vi "GetAllWatchdogs.vi"(8 "error in (no error)":errorcluster, 11 "Pound in":refnum<class "Pound.lvclass">) -> (0 "error out":errorcluster, 2 "All Watchdogs":refnum<data-value>[](array[refnum]), 3 "Pound out":refnum<class "Pound.lvclass">)   [LabVIEW 2017, in "Pound.lvclass"]
uses:
  <vilib>/NI/Software Watchdog/Pound/Pound.lvclass
  <vilib>/NI/Software Watchdog/Watchdog/Watchdog.lvclass
  <vilib>/NI/Software Watchdog/Pound/Pound.lvclass/Pound.ctl
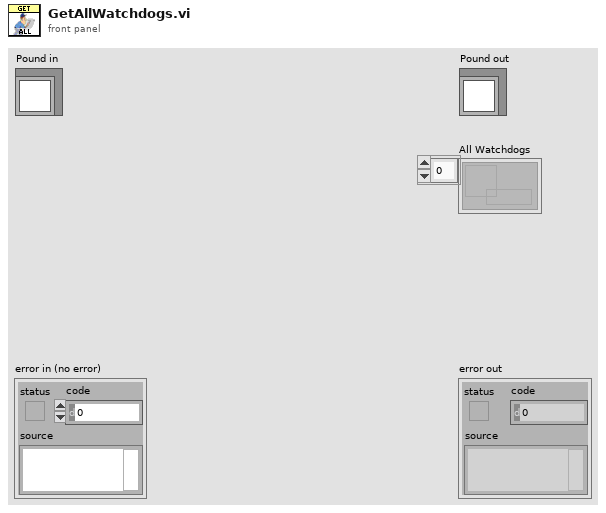
[diagram p1: front panel]
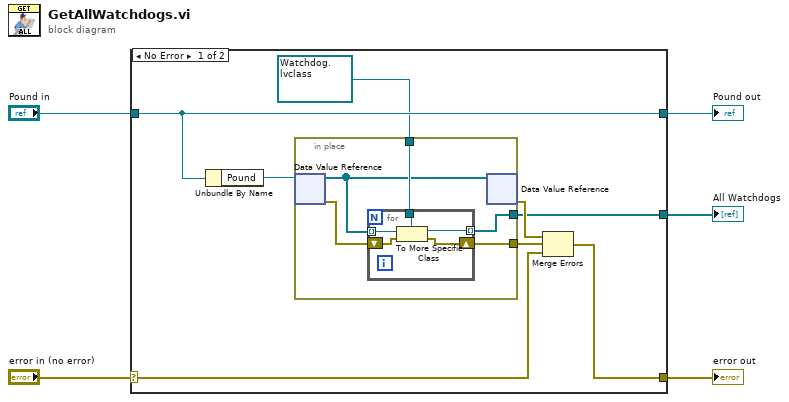
[diagram p0: block diagram]
diagram:
  n1 = case shown="No Error" "error in (no error)" {
    selector: "error in (no error)" -> [w6 w25]
    tunnel: [w8 w25] -> w4
    tunnel: [w12 w24] -> w2
    tunnel: "Pound in" -> [w12 w24]
    tunnel: [w7 _] -> w1
    frame No Error {
      n2 = Unbundle By Name(w12) -> ("Pound"=w13:refnum<data-value>)
      n3 = in-place {
        in-place-border: refnum<data-value> refnum ("data value reference") -> [w18]
        in-place-border: [w15] -> w9
        in-place-border: [w14] -> w7
        n4 = in-place-dvr #1(w13) -> (w16:refnum<data-value>[], w17:errorcluster)
        n5 = for {
          tunnel: w16 -> [w23] mode=indexing
          tunnel: w18 -> [w22]
          tunnel: [w21] -> w14 mode=indexing
          shift-right: [w20] -> w15
          shift-left: w17 -> [w19]
          n6 = To More Specific Class(target class=w22, reference=w23, error in=w19) -> (specific class reference=w21:refnum<data-value>, error out=w20:errorcluster)
        }
        n7 = in-place-dvr #1(w16) -> (w10:errorcluster)  [unwired: 1 out]
      }
      n8 = Merge Errors(w10, w9, w6) -> (w8:errorcluster)
    }
    frame Error {
    }
  }
  "error out" <- w4
  "Pound out" <- w2
  "All Watchdogs" <- w1
